vi "LabviewProjectWorkingDisplay.vi"() -> ()   [LabVIEW 2025]
panel:
  out "x = y? 2":bool
  out "x = y?":bool
  out "Array":dbl[](array[numeric])
  out "Boolean":bool
  in  "SPIN":bool
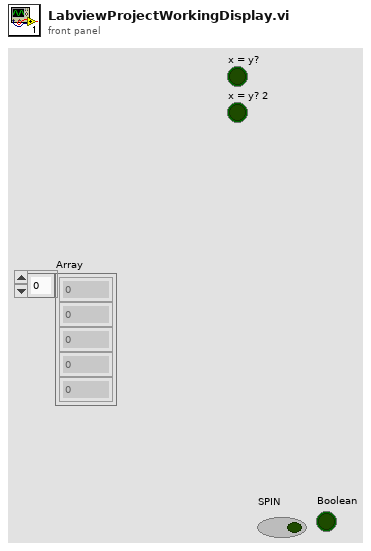
[diagram p1: front panel]
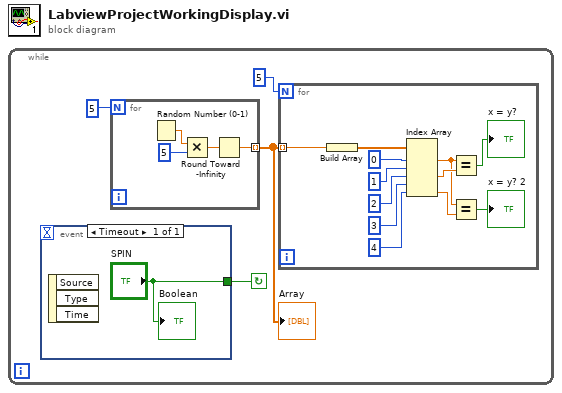
[diagram p0: block diagram]
diagram:
  n1 = while {
    stop <- w4 continue-if-true
    n2 = event shown="[0] Timeout" {
      selector: _ -> [_]
      dyn-events: _ -> [_]
      timeout: _ -> [_]
      tunnel: ["SPIN"] -> w4
      event Timeout {
        n3 = event-data() -> ()  [unwired: 1 in, 3 out]
        "Boolean" <- "SPIN"
      }
    }
    n4 = for {
      N: 5 -> [_]
      tunnel: [w17] -> w2 mode=indexing
      n5 = Random Number (0-1)() -> (number: 0 to 1=w20:dbl)
      n6 = Multiply(x=w20, y=5) -> (x*y=w18:dbl)
      n7 = Round Toward -Infinity(1:w18) -> (0:w17:dbl)
    }
    "Array" <- w2
    n8 = for {
      N: 5 -> [_]
      tunnel: w2 -> [w16] mode=indexing
      n9 = Build Array(w16) -> (w15:dbl[])
      n10 = Index Array(array=w15, index #1=0, index #2=1, index #3=2, index #4=3, index #5=4) -> (element #1=w12:dbl, element #3=w14:dbl, element #5=w13:dbl)  [unwired: 2 out]
      n11 = Equal?(x=w12, y=w14) -> (x = y?=→"x = y?":bool)
      n12 = Equal?(x=w12, y=w13) -> (x = y?=→"x = y? 2":bool)
    }
  }
